vi "Index Array Function.vi"() -> ()   [LabVIEW 2012]
panel:
  out "Extracted Column":i32[](array[numeric])
  out "Extracted Element":i32
  out "Extracted Row":i32[](array[numeric])
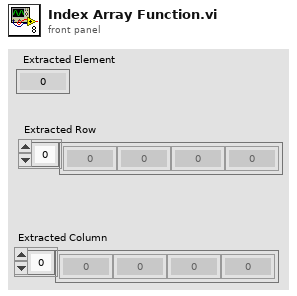
[diagram p1: front panel]
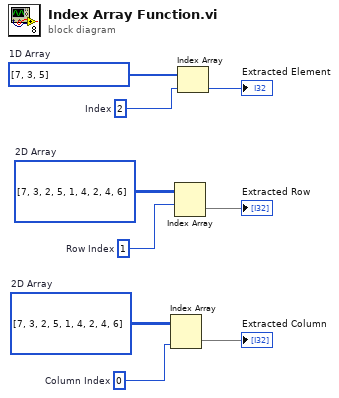
[diagram p0: block diagram]
diagram:
  w1 = 0  # Column Index
  w2 = i32[][] [[7, 3, 2], [5, 1, 4], [2, 4, 6]]  # 2D Array
  w6 = 1  # Row Index
  w7 = i32[][] [[7, 3, 2], [5, 1, 4], [2, 4, 6]]  # 2D Array
  w8 = 2  # Index
  w9 = i32[] [7, 3, 5]  # 1D Array
  n1 = Index Array "Index Array"(array=w2, index (col)=w1) -> (element=→"Extracted Column":i32[])  [unwired: 1 in]
  n2 = Index Array "Index Array"(array=w7, index (row)=w6) -> (element=→"Extracted Row":i32[])  [unwired: 1 in]
  n3 = Index Array "Index Array"(array=w9, index=w8) -> (element=→"Extracted Element":i32)
